vi "execution class name.vi"(8 "error in":errorcluster, 11 "ExampleSequencer configuration in":refnum<class "ExampleSequencer configuration.lvclass">) -> (0 "error out":errorcluster, 2 "class name":string, 3 "ExampleSequencer configuration out":refnum<class "ExampleSequencer configuration.lvclass">)   [LabVIEW 2017, in "ExampleSequencer configuration.lvclass"]
doc: "Provides an interface for determining the module runtime class associated with this module configuration. This class name can then be used to dynamically load or locate the runtime class for initialization purposes."
uses:
  ExampleSequencer configuration.lvclass
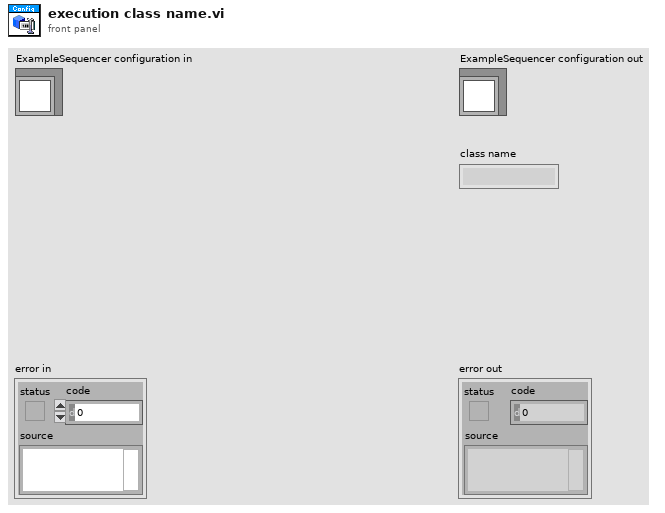
[diagram p1: front panel]
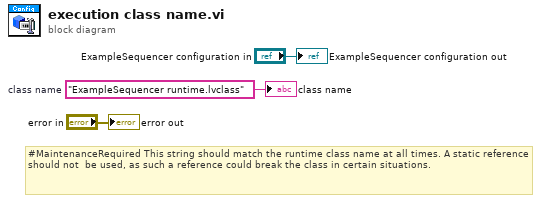
[diagram p0: block diagram]
diagram:
  w1 = "ExampleSequencer runtime.lvclass"  # class name
  # "#MaintenanceRequired This string should match the runtime class name at all times. A static reference should not  be used, as such a reference could break the class in certain situations."
  "error out" <- "error in"
  "ExampleSequencer configuration out" <- "ExampleSequencer configuration in"
  "class name" <- w1
